vi "Mask XY Graph.vi"(8 "error in (no error)":errorcluster, 10 "Mask":cluster{"X":dbl[], "Y":dbl[]}, 11 "Data":cluster{"X":dbl[], "Y":dbl[]}) -> (0 "error out":errorcluster, 2 "Unmasked Data":cluster{"X":dbl[], "Y":dbl[]}, 3 "Masked Data":cluster{"X":dbl[], "Y":dbl[]})   [LabVIEW 2023]
doc: "Given a data set and a mask, generate XY arrays for the masked data and the unmasked data."
uses:
  <vilib>/Analysis/geometry.llb/Point in Polygon Position.ctl
  <vilib>/Utility/error.llb/Error Cluster From Error Code.vi
  <vilib>/Analysis/geometry.llb/Point in Polygon (Scalar).vi
  <vilib>/ErrorRing/Error Ring.xnode
  <vilib>/Analysis/NI_AAL_Geometry.lvlib
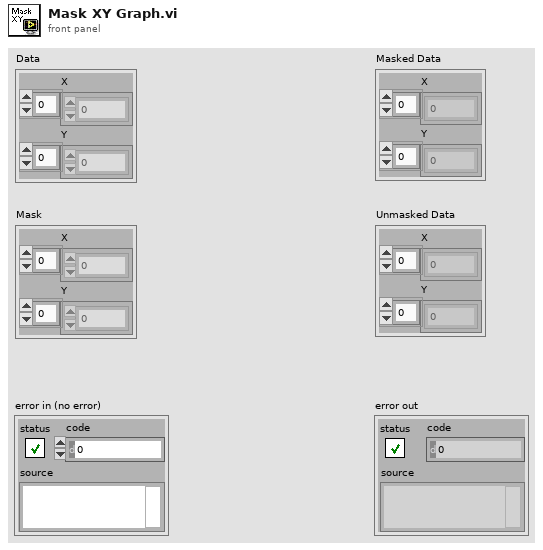
[diagram p1: front panel]
types:
  T1 = typedef "NI_AAL_Geometry.lvlib/Point in Polygon Position.ctl" = u16
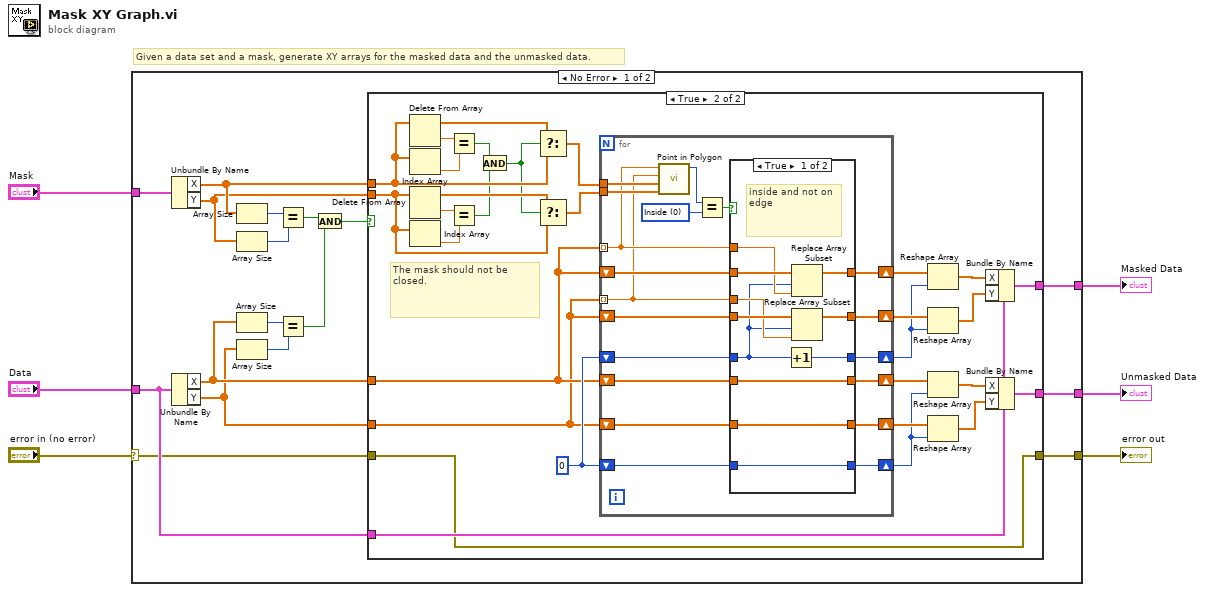
[diagram p0: block diagram]
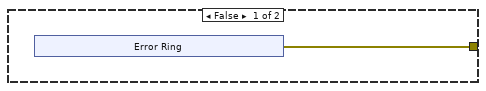
[diagram p2: hidden frame]
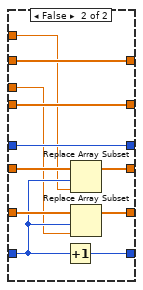
[diagram p3: hidden frame]
diagram:
  # "Given a data set and a mask, generate XY arrays for the masked data and the unmasked data."
  n1 = case shown="No Error" "error in (no error)" {
    selector: "error in (no error)" -> [w7 w100]
    tunnel: "Mask" -> [w23 _]
    tunnel: "Data" -> [w22 _]
    tunnel: [w21 _] -> w4
    tunnel: [w20 _] -> w3
    tunnel: [w8 w100] -> w1
    frame No Error {
      n2 = Unbundle By Name(w23) -> ("X"=w19:dbl[], "Y"=w18:dbl[])
      n3 = Unbundle By Name(w22) -> ("X"=w17:dbl[], "Y"=w16:dbl[])
      n4 = Array Size(array=w19) -> (size(s)=w15:i32)
      n5 = Array Size(array=w18) -> (size(s)=w14:i32)
      n6 = Array Size(array=w17) -> (size(s)=w13:i32)
      n7 = Array Size(array=w16) -> (size(s)=w12:i32)
      n8 = Equal?(x=w15, y=w14) -> (x = y?=w11:bool)
      n9 = Equal?(x=w13, y=w12) -> (x = y?=w10:bool)
      n10 = And(x=w11, y=w10) -> (x .and. y?=w9:bool)
      n11 = case shown="True" w9 {
        tunnel: w22 -> [_ w48]
        tunnel: [_ w47] -> w21
        tunnel: [_ w46] -> w20
        tunnel: w19 -> [_ w37]
        tunnel: w18 -> [_ w35]
        tunnel: w17 -> [_ w38]
        tunnel: w16 -> [_ w33]
        tunnel: [w24 w29] -> w8
        tunnel: w7 -> [_ w29]
        frame False {
          n12 = xnode "Error Ring"() -> ("error out"=w24:errorcluster)
        }
        frame True {
          w55 = 0
          # "The mask should not be closed."
          n13 = Delete From Array(array=w37) -> (deleted portion=w44:dbl, array with subset deleted=w42:dbl[])  [unwired: 2 in]
          n14 = Index Array(array=w37) -> (element=w43:dbl)  [unwired: 1 in]
          n15 = Delete From Array(array=w35) -> (deleted portion=w39:dbl, array with subset deleted=w41:dbl[])  [unwired: 2 in]
          n16 = Index Array(array=w35) -> (element=w40:dbl)  [unwired: 1 in]
          n17 = Equal?(x=w44, y=w43) -> (x = y?=w32:bool)
          n18 = Equal?(x=w39, y=w40) -> (x = y?=w31:bool)
          n19 = And(x=w32, y=w31) -> (x .and. y?=w30:bool)
          n20 = Select(t=w42, s=w30, f=w37) -> (s? t:f=w36:dbl[])
          n21 = Select(t=w41, s=w30, f=w35) -> (s? t:f=w34:dbl[])
          n22 = for {
            tunnel: w36 -> [w65]
            tunnel: w34 -> [w64]
            tunnel: w38 -> [w63] mode=indexing
            tunnel: w33 -> [w62] mode=indexing
            shift-right: [w74] -> w57
            shift-left: w33 -> [w76]
            shift-right: [w75] -> w58
            shift-left: w38 -> [w77]
            shift-right: [w72] -> w56
            shift-left: w55 -> [w73]
            shift-right: [w68] -> w53
            shift-left: w33 -> [w69]
            shift-right: [w70] -> w54
            shift-left: w38 -> [w71]
            shift-right: [w66] -> w52
            shift-left: w55 -> [w67]
            w60 = T1 0 items=["Inside", "On Boundary", "Outside"] ("position")
            n23 = call-poly <vilib>:"Point in Polygon.vi"("Polygon Y"=w64, "Polygon X"=w65, "y"=w62, "x"=w63) -> ("position"=w61:T1)  [unwired: 6 in, 1 out]
            n24 = Equal?(x=w61, y=w60) -> (x = y?=w59:bool)
            n25 = case shown="True" w59 {
              tunnel: w63 -> [w87 w90]
              tunnel: w77 -> [w88 w99]
              tunnel: w62 -> [w85 w89]
              tunnel: w76 -> [w86 w98]
              tunnel: [w84 w99] -> w75
              tunnel: [w83 w98] -> w74
              tunnel: w73 -> [w82 w97]
              tunnel: [w81 w97] -> w72
              tunnel: w71 -> [w80 w96]
              tunnel: [w80 w95] -> w70
              tunnel: w69 -> [w79 w94]
              tunnel: [w79 w93] -> w68
              tunnel: w67 -> [w78 w92]
              tunnel: [w78 w91] -> w66
              frame True {
                # "inside and not on edge"
                n26 = Increment(x=w82) -> (x+1=w81:i32)
                n27 = Replace Array Subset(array=w88, new element=w87, index=w82) -> (w84:dbl[])
                n28 = Replace Array Subset(array=w86, new element=w85, index=w82) -> (w83:dbl[])
              }
              frame False {
                n29 = Increment(x=w92) -> (x+1=w91:i32)
                n30 = Replace Array Subset(array=w96, new element=w90, index=w92) -> (w95:dbl[])
                n31 = Replace Array Subset(array=w94, new element=w89, index=w92) -> (w93:dbl[])
              }
            }
          }
          n32 = Reshape Array(w58, w56) -> (w51:dbl[])
          n33 = Reshape Array(w57, w56) -> (w50:dbl[])
          n34 = Reshape Array(w54, w52) -> (w49:dbl[])
          n35 = Reshape Array(w53, w52) -> (w45:dbl[])
          n36 = Bundle By Name(cluster=w48, "X"=w51, "Y"=w50) -> (w47:cluster{"X":dbl[], "Y":dbl[]})
          n37 = Bundle By Name(cluster=w48, "X"=w49, "Y"=w45) -> (w46:cluster{"X":dbl[], "Y":dbl[]})
        }
      }
    }
    frame Error {
    }
  }
  "Unmasked Data" <- w3
  "Masked Data" <- w4
  "error out" <- w1
